vi "Read Raw Data.vi"(7 "SR Creation Date Range":T1, 8 "Error In":errorcluster, 9 "Employees":string[](array[string]), 10 "Countries":string[](array[string]), 11 "DVR In":refnum<data-value>) -> (0 "Error Out":errorcluster, 2 "data value reference":refnum<data-value>, 3 "DVR Out":refnum<data-value>, 5 "Elements Found":i32)   [LabVIEW 2016, in "Data Operations.lvlib"]
uses:
  Data Operations.lvlib
  Private Controls/Report Data Cluster.ctl
  Private Controls/Data Raw.ctl
  Public Controls/Start End Date Cluster.ctl
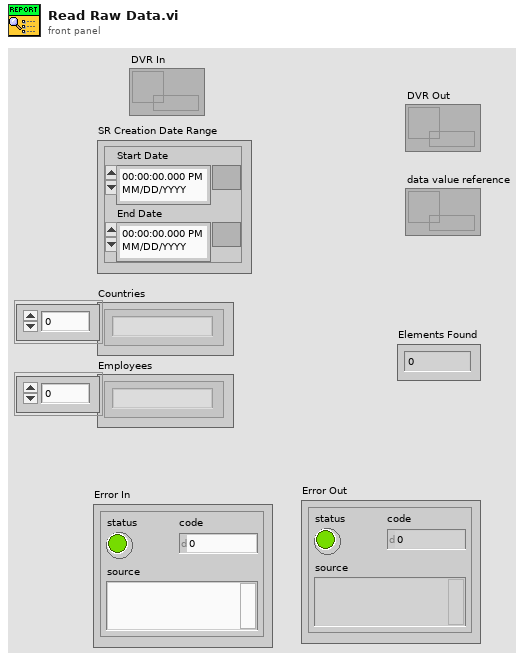
[diagram p1: front panel]
types:
  T1 = typedef "Data Operations.lvlib/Start End Date Cluster.ctl" = cluster{"Start Date":timestamp, "End Date":timestamp}
  T2 = typedef "Data Operations.lvlib/Report Data Cluster.ctl" = cluster{"Headers":cluster{"Start Date":timestamp, "End Date":timestamp, "SR Status String":string[], "AE Owner String":string[]}, "Data":T3[]}
  T3 = typedef "Data Operations.lvlib/Data Raw.ctl" = cluster{"SR Number":string, "Status":string, "Summary":string, "AE Owner":string, "AE Group":string, "SurveyData":cluster{"Resolution Time":dbl, "Total Satisfaction":dbl, "Response Time":dbl, "Courtesy":dbl, "Problem Solved":dbl}, "Time Data":cluster{"Last Update Date":timestamp, "Request Date":timestamp, "Request week":u8}}
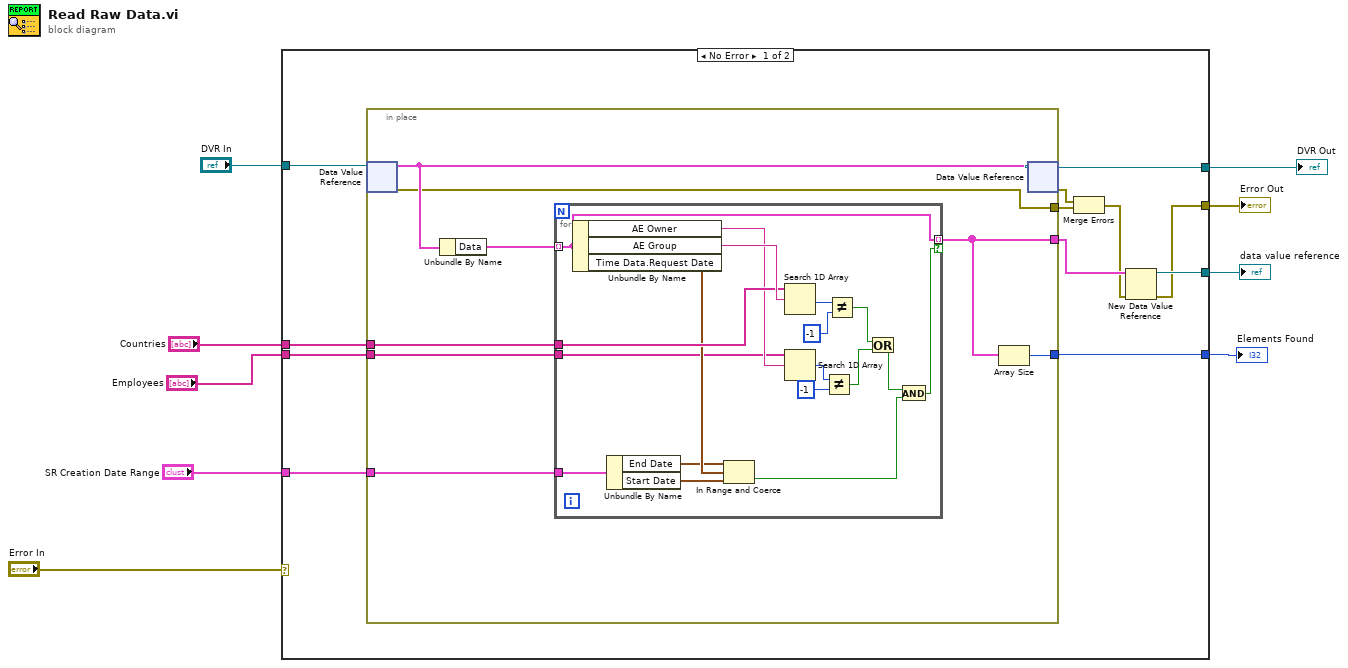
[diagram p0: block diagram]
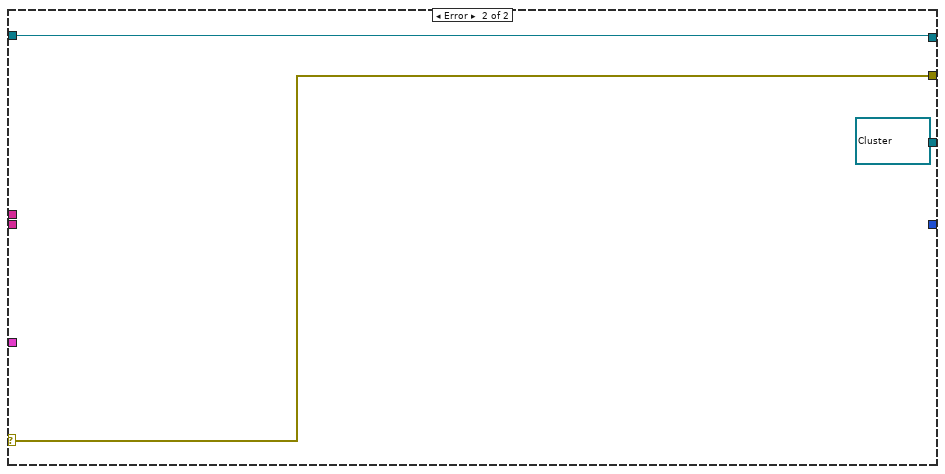
[diagram p2: hidden frame]
diagram:
  n1 = case shown="No Error" "Error In" {
    selector: "Error In" -> [_ w50]
    tunnel: "DVR In" -> [w21 w49]
    tunnel: [w12 w50] -> w8
    tunnel: [w18 w49] -> w7
    tunnel: "Countries" -> [w17 _]
    tunnel: "Employees" -> [w16 _]
    tunnel: [w14 refnum<data-value> refnum ("data value reference")] -> w3
    tunnel: [w11 _] -> w2
    tunnel: "SR Creation Date Range" -> [w10 _]
    frame No Error {
      n2 = in-place {
        in-place-border: [w28] -> w19
        in-place-border: w17 -> [w26]
        in-place-border: w16 -> [w25]
        in-place-border: [w24] -> w15
        in-place-border: [w23] -> w11
        in-place-border: w10 -> [w22]
        n3 = in-place-dvr #1(w21) -> (w29:T2, w28:errorcluster)
        n4 = Unbundle By Name(w29) -> ("Data"=w27:T3[])
        n5 = for {
          tunnel: w27 -> [w40] mode=indexing
          tunnel: w26 -> [w46]
          tunnel: w25 -> [w32]
          tunnel: [w40] -> w24 mode=indexing if=w31
          tunnel: w22 -> [w39]
          n6 = Unbundle By Name(w40) -> ("AE Owner"=w33:string, "AE Group"=w47:string, "Time Data.Request Date"=w38:timestamp)
          n7 = Unbundle By Name(w39) -> ("End Date"=w37:timestamp, "Start Date"=w36:timestamp)
          n8 = In Range and Coerce(upper limit=w37, x=w38, lower limit=w36) -> (In Range?=w30:bool)  [unwired: 1 out]
          n9 = Search 1D Array(1D array=w46, element=w47) -> (index of element=w45:i32)  [unwired: 1 in]
          n10 = Search 1D Array(1D array=w32, element=w33) -> (index of element=w44:i32)  [unwired: 1 in]
          n11 = Not Equal?(x=w44, y=-1) -> (x != y?=w34:bool)
          n12 = Not Equal?(x=w45, y=-1) -> (x != y?=w41:bool)
          n13 = Or(x=w41, y=w34) -> (x .or. y?=w35:bool)
          n14 = And(x=w35, y=w30) -> (x .and. y?=w31:bool)
        }
        n15 = Array Size(array=w24) -> (size(s)=w23:i32)
        n16 = in-place-dvr #1(w29) -> (w18:refnum<data-value>, w20:errorcluster)
      }
      n17 = Merge Errors(w20, w19) -> (w13:errorcluster)
      n18 = New Data Value Reference(data value=w15, error in=w13) -> (data value reference=w14:refnum<data-value>, error out=w12:errorcluster)
    }
    frame Error {
    }
  }
  "Error Out" <- w8
  "DVR Out" <- w7
  "data value reference" <- w3
  "Elements Found" <- w2
